vi "release file IO queue.vi"(11 "Queues":T1) -> ()   [LabVIEW 2018]
uses:
  type defs/Queues.ctl
types:
  T1 = typedef "Queues.ctl" = cluster{"messageHandler":refnum<queue>, "comms":refnum<queue>, "dataStream":refnum<queue>, "dataProcessor":refnum<queue>, "fileIO":refnum<queue>, "userInterface":refnum<queue>, "errors":refnum<queue>, "customCompressor":refnum<queue>}
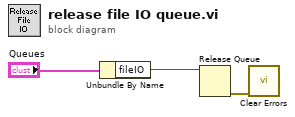
[diagram p0: block diagram]
diagram:
  n1 = Unbundle By Name("Queues") -> ("fileIO"=w2:refnum<queue>)
  n2 = Release Queue(queue=w2) -> (error out=w1:errorcluster)  [unwired: 2 in, 2 out]
  n3 = call <vilib>:"Clear Errors.vi"("error in (no error)"=w1) -> ()  [unwired: 5 in, 2 out]
